vi "E727_StageNavigatorModule.vi"(0 "Up Z x4":bool, 1 "Up Z x2":bool, 2 "Up Z":bool, 3 "StageChannels":string[](array[string]), 4 "Up x4":bool, 5 "Up x2":bool, 6 "Up":bool, 7 "Up x0.5":bool, 8 "Right x0.5":bool, 9 "Left x0.5":bool, 10 "Right":bool, 11 "Left":bool, 12 "Right x2":bool, 13 "Left x2":bool, 14 "Right x4":bool, 15 "Left x4":bool, 17 "X / Y Resolution (um)":dbl=10.0 min=1.0, 19 "Z Resolution (um)":dbl=30.0 min=1.0, 20 "Down Z x4":bool, 21 "Down Z x2":bool, 22 "Down Z":bool, 23 "stop":bool, 24 "Down x4":bool, 25 "Down x2":bool, 26 "Down":bool, 27 "Down x0.5":bool) -> (16 "Position":dbl[](array[numeric]) format="%.6f")   [LabVIEW 2022 SP3]
panel:
  in  "Repeats":dbl=1.0 min=1.0
  # "STAGE"
  # "Z Focus"
  # "X / Y Navigation"
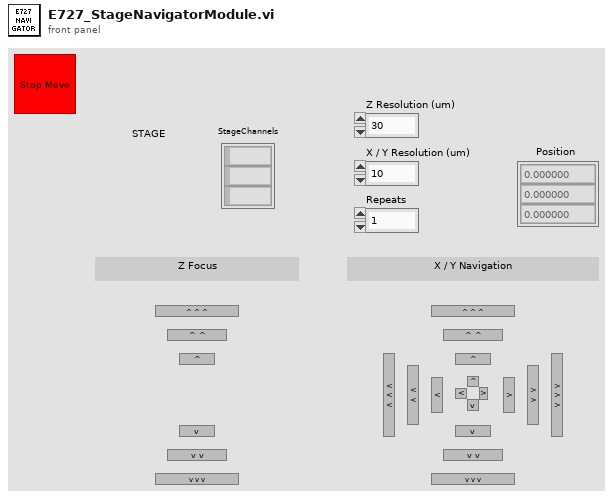
[diagram p1: front panel]
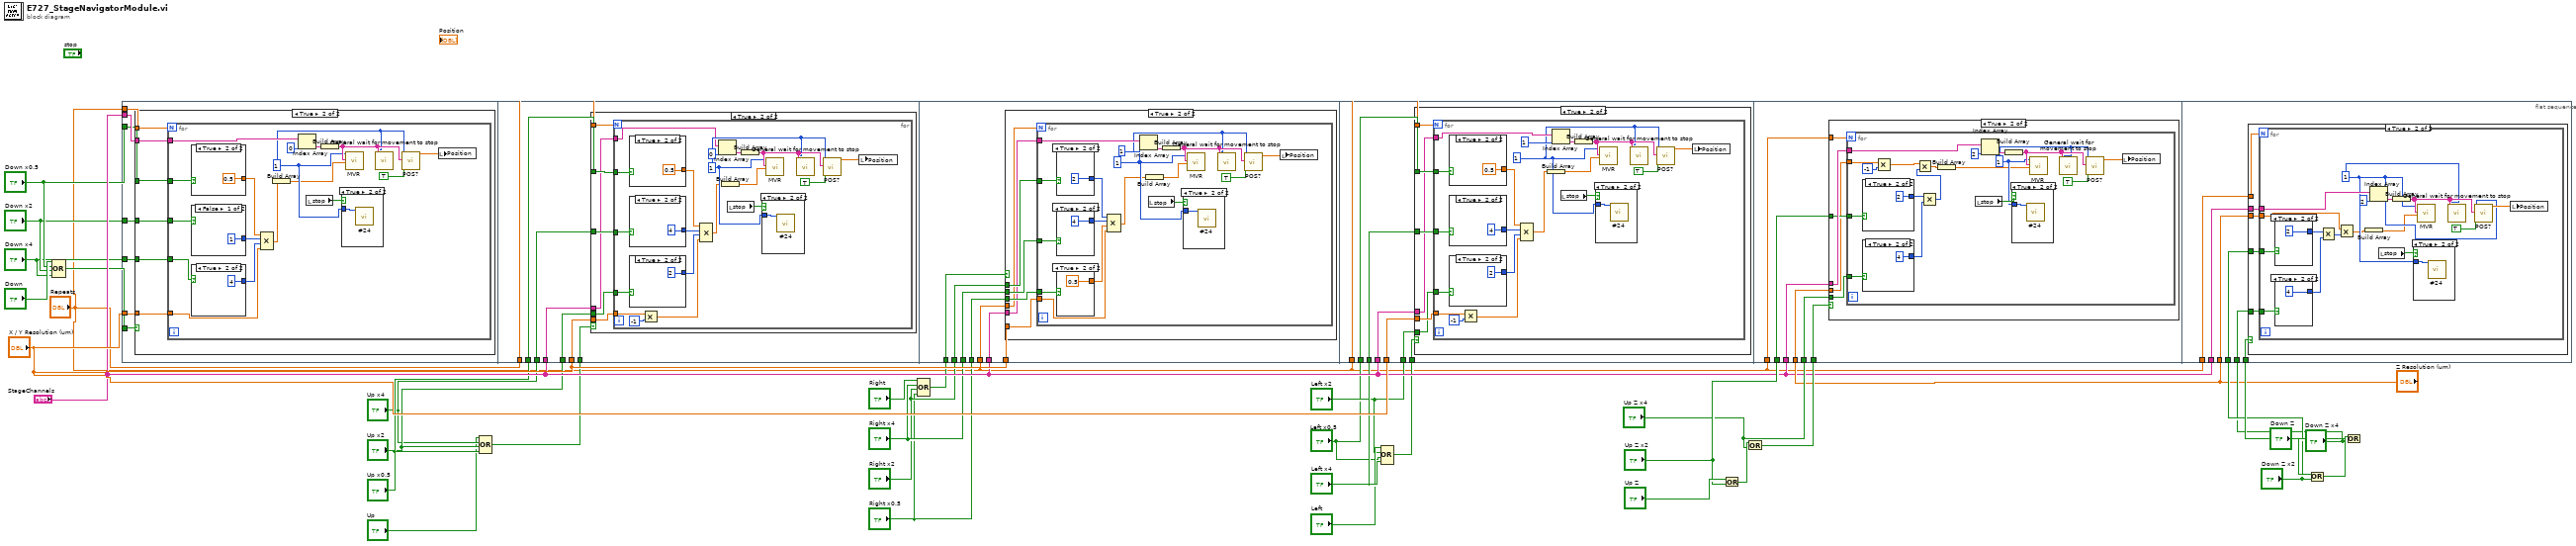
[diagram p0: block diagram]
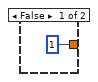
[diagram p4: hidden frame]
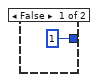
[diagram p5: hidden frame]
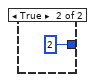
[diagram p6: hidden frame]
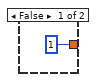
[diagram p9: hidden frame]
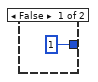
[diagram p10: hidden frame]
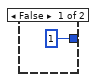
[diagram p11: hidden frame]
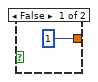
[diagram p14: hidden frame]
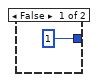
[diagram p15: hidden frame]
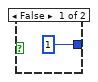
[diagram p16: hidden frame]
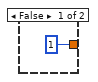
[diagram p19: hidden frame]
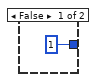
[diagram p20: hidden frame]
diagram:
  n1 = Compound Arithmetic op=OR("Down", "Down x0.5", "Down x2", "Down x4") -> (w6:bool)
  n2 = flat-sequence {
    tunnel: "X / Y Resolution (um)" -> [w40]
    tunnel: "StageChannels" -> [w41]
    tunnel: w6 -> [w39]
    tunnel: "Down x2" -> [w38]
    tunnel: "Down x4" -> [w37]
    tunnel: "Down x0.5" -> [w36]
    tunnel: "Repeats" -> [w35]
    tunnel: "X / Y Resolution (um)" -> [w78]
    tunnel: "StageChannels" -> [w77]
    tunnel: "Up x2" -> [w76]
    tunnel: w11 -> [w75]
    tunnel: "Up x4" -> [w74]
    tunnel: "Up x0.5" -> [w73]
    tunnel: "Repeats" -> [w72]
    tunnel: "StageChannels" -> [w117]
    tunnel: "Right x2" -> [w116]
    tunnel: "Right x4" -> [w115]
    tunnel: "X / Y Resolution (um)" -> [w114]
    tunnel: w21 -> [w113]
    tunnel: "Right x0.5" -> [w112]
    tunnel: "Repeats" -> [w111]
    tunnel: "StageChannels" -> [w154]
    tunnel: "X / Y Resolution (um)" -> [w153]
    tunnel: w16 -> [w152]
    tunnel: "Left x4" -> [w151]
    tunnel: "Left x2" -> [w150]
    tunnel: "Left x0.5" -> [w149]
    tunnel: "Repeats" -> [w148]
    tunnel: "StageChannels" -> [w192]
    tunnel: "Z Resolution (um)" -> [w191]
    tunnel: w32 -> [w190]
    tunnel: "Up Z x2" -> [w189]
    tunnel: "Up Z x4" -> [w188]
    tunnel: "Repeats" -> [w187]
    tunnel: "StageChannels" -> [w226]
    tunnel: "Z Resolution (um)" -> [w225]
    tunnel: w26 -> [w224]
    tunnel: "Down Z x2" -> [w223]
    tunnel: "Down Z x4" -> [w222]
    tunnel: "Repeats" -> [w221]
    frame #0 {
      n3 = case shown="True" w39 {
        tunnel: w40 -> [_ w44]
        tunnel: w41 -> [_ w47]
        tunnel: w38 -> [_ w46]
        tunnel: w37 -> [_ w45]
        tunnel: w36 -> [_ w43]
        tunnel: w35 -> [_ w42]
        frame False {
        }
        frame True {
          n4 = for {
            N: w42 -> [_]
            tunnel: w47 -> [w51]
            tunnel: w46 -> [w64]
            tunnel: w45 -> [w63]
            tunnel: w44 -> [w62]
            tunnel: w43 -> [w58]
            w50 = 1 ("System no.")
            n5 = case shown="True" w58 {
              tunnel: [1 0.5] -> w61
              frame False {
              }
              frame True {
              }
            }
            n6 = case shown="False" w64 {
              tunnel: [1 2] -> w59
              frame False {
              }
              frame True {
              }
            }
            n7 = case shown="True" w63 {
              tunnel: [1 4] -> w60
              frame False {
              }
              frame True {
              }
            }
            n8 = Compound Arithmetic op=MULTIPLY(w61, w59, w60, w62) -> (w49:dbl)
            n9 = Build Array(w49) -> (w48:dbl[])
            n10 = Index Array(array=w51, index=0) -> (element=w54:string)
            n11 = local read "stop"() -> (w55:bool)
            n12 = Build Array(w54) -> (w56:string[])
            n13 = case shown="True" w55 {
              tunnel: w50 -> [_ w65]
              frame False {
              }
              frame True {
                n14 = call "#24.vi"("System no."=w65) -> ()  [unwired: 1 in, 18 out]
              }
            }
            n15 = call "MVR.vi"("System no."=w50, "Axes to move"=w56, "Position values"=w48) -> ()  [unwired: 2 in, 15 out]
            n16 = call "General wait for movement to stop.vi"("System no."=w50, "Axes to wait for"=w56) -> ()  [unwired: 6 in, 12 out]
            n17 = call "POS?.vi"("System no."=w50, "Axes to query"=w56, "All axes?"=TRUE) -> ("Position"=w57:dbl[])  [unwired: 2 in, 14 out]
            n18 = local write "Position"(w57) -> ()
          }
        }
      }
    }
    frame #1 {
      n19 = case shown="True" w75 {
        tunnel: w78 -> [_ w84]
        tunnel: w77 -> [_ w80]
        tunnel: w76 -> [_ w83]
        tunnel: w74 -> [_ w82]
        tunnel: w73 -> [_ w81]
        tunnel: w72 -> [_ w79]
        frame False {
        }
        frame True {
          n20 = for {
            N: w79 -> [_]
            tunnel: w84 -> [w95]
            tunnel: w83 -> [w102]
            tunnel: w82 -> [w101]
            tunnel: w81 -> [w96]
            tunnel: w80 -> [w87]
            w88 = 1 ("System no.")
            n21 = case shown="True" w96 {
              tunnel: [1 0.5] -> w99
              frame False {
              }
              frame True {
              }
            }
            n22 = case shown="True" w101 {
              tunnel: [1 4] -> w98
              frame False {
              }
              frame True {
              }
            }
            n23 = case shown="True" w102 {
              tunnel: [1 2] -> w97
              frame False {
              }
              frame True {
              }
            }
            n24 = Multiply(x=w95, y=-1) -> (x*y=w100:dbl)
            n25 = Compound Arithmetic op=MULTIPLY(w99, w98, w97, w100) -> (w85:dbl)
            n26 = Index Array(array=w87, index=0) -> (element=w91:string)
            n27 = Build Array(w85) -> (w86:dbl[])
            n28 = local read "stop"() -> (w92:bool)
            n29 = Build Array(w91) -> (w93:string[])
            n30 = case shown="True" w92 {
              tunnel: w88 -> [_ w104]
              frame False {
              }
              frame True {
                n31 = call "#24.vi"("System no."=w104) -> ()  [unwired: 1 in, 18 out]
              }
            }
            n32 = call "MVR.vi"("System no."=w88, "Axes to move"=w93, "Position values"=w86) -> ()  [unwired: 2 in, 15 out]
            n33 = call "General wait for movement to stop.vi"("System no."=w88, "Axes to wait for"=w93) -> ()  [unwired: 6 in, 12 out]
            n34 = call "POS?.vi"("System no."=w88, "Axes to query"=w93, "All axes?"=TRUE) -> ("Position"=w94:dbl[])  [unwired: 2 in, 14 out]
            n35 = local write "Position"(w94) -> ()
          }
        }
      }
    }
    frame #2 {
      n36 = case shown="True" w113 {
        tunnel: w114 -> [_ w120]
        tunnel: w117 -> [_ w119]
        tunnel: w116 -> [_ w123]
        tunnel: w115 -> [_ w122]
        tunnel: w112 -> [_ w121]
        tunnel: w111 -> [_ w118]
        frame False {
        }
        frame True {
          n37 = for {
            N: w118 -> [_]
            tunnel: w123 -> [w140]
            tunnel: w122 -> [w139]
            tunnel: w121 -> [w137]
            tunnel: w120 -> [w134]
            tunnel: w119 -> [w128]
            w126 = 1 ("System no.")
            n38 = case shown="True" w140 {
              tunnel: [1 2] -> w136
              frame False {
              }
              frame True {
              }
            }
            n39 = case shown="True" w139 {
              tunnel: [1 4] -> w135
              frame False {
              }
              frame True {
              }
            }
            n40 = case shown="True" w137 {
              tunnel: [1 0.5] -> w138
              frame False {
              }
              frame True {
              }
            }
            n41 = Compound Arithmetic op=MULTIPLY(w136, w135, w138, w134) -> (w124:dbl)
            n42 = Index Array(array=w128, index=1) -> (element=w130:string)
            n43 = Build Array(w124) -> (w125:dbl[])
            n44 = local read "stop"() -> (w131:bool)
            n45 = Build Array(w130) -> (w132:string[])
            n46 = case shown="True" w131 {
              tunnel: w126 -> [_ w141]
              frame False {
              }
              frame True {
                n47 = call "#24.vi"("System no."=w141) -> ()  [unwired: 1 in, 18 out]
              }
            }
            n48 = call "MVR.vi"("System no."=w126, "Axes to move"=w132, "Position values"=w125) -> ()  [unwired: 2 in, 15 out]
            n49 = call "General wait for movement to stop.vi"("System no."=w126, "Axes to wait for"=w132) -> ()  [unwired: 6 in, 12 out]
            n50 = call "POS?.vi"("System no."=w126, "Axes to query"=w132, "All axes?"=TRUE) -> ("Position"=w133:dbl[])  [unwired: 2 in, 14 out]
            n51 = local write "Position"(w133) -> ()
          }
        }
      }
    }
    frame #3 {
      n52 = case shown="True" w152 {
        tunnel: w153 -> [_ w160]
        tunnel: w154 -> [_ w156]
        tunnel: w150 -> [_ w159]
        tunnel: w151 -> [_ w158]
        tunnel: w149 -> [_ w157]
        tunnel: w148 -> [_ w155]
        frame False {
        }
        frame True {
          n53 = for {
            N: w155 -> [_]
            tunnel: w160 -> [w179]
            tunnel: w159 -> [w177]
            tunnel: w158 -> [w176]
            tunnel: w157 -> [w171]
            tunnel: w156 -> [w164]
            w163 = 1 ("System no.")
            n54 = case shown="True" w171 {
              tunnel: [1 0.5] -> w175
              frame False {
              }
              frame True {
              }
            }
            n55 = case shown="True" w176 {
              tunnel: [1 4] -> w173
              frame False {
              }
              frame True {
              }
            }
            n56 = case shown="True" w177 {
              tunnel: [1 2] -> w172
              frame False {
              }
              frame True {
              }
            }
            n57 = Multiply(x=w179, y=-1) -> (x*y=w174:dbl)
            n58 = Compound Arithmetic op=MULTIPLY(w175, w173, w172, w174) -> (w161:dbl)
            n59 = Build Array(w161) -> (w162:dbl[])
            n60 = Index Array(array=w164, index=1) -> (element=w167:string)
            n61 = local read "stop"() -> (w168:bool)
            n62 = Build Array(w167) -> (w169:string[])
            n63 = case shown="True" w168 {
              tunnel: w163 -> [_ w180]
              frame False {
              }
              frame True {
                n64 = call "#24.vi"("System no."=w180) -> ()  [unwired: 1 in, 18 out]
              }
            }
            n65 = call "MVR.vi"("System no."=w163, "Axes to move"=w169, "Position values"=w162) -> ()  [unwired: 2 in, 15 out]
            n66 = call "General wait for movement to stop.vi"("System no."=w163, "Axes to wait for"=w169) -> ()  [unwired: 6 in, 12 out]
            n67 = call "POS?.vi"("System no."=w163, "Axes to query"=w169, "All axes?"=TRUE) -> ("Position"=w170:dbl[])  [unwired: 2 in, 14 out]
            n68 = local write "Position"(w170) -> ()
          }
        }
      }
    }
    frame #4 {
      n69 = case shown="True" w190 {
        tunnel: w191 -> [_ w194]
        tunnel: w192 -> [_ w197]
        tunnel: w189 -> [_ w196]
        tunnel: w188 -> [_ w195]
        tunnel: w187 -> [_ w193]
        frame False {
        }
        frame True {
          n70 = for {
            N: w193 -> [_]
            tunnel: w197 -> [w201]
            tunnel: w196 -> [w212]
            tunnel: w195 -> [w211]
            tunnel: w194 -> [w208]
            w200 = 1 ("System no.")
            n71 = case shown="True" w212 {
              tunnel: [1 2] -> w214
              frame False {
              }
              frame True {
              }
            }
            n72 = case shown="True" w211 {
              tunnel: [1 4] -> w215
              frame False {
              }
              frame True {
              }
            }
            n73 = Multiply(x=w208, y=-1) -> (x*y=w209:dbl)
            n74 = Multiply(x=w214, y=w215) -> (x*y=w213:i32)
            n75 = Multiply(x=w209, y=w213) -> (x*y=w199:dbl)
            n76 = Build Array(w199) -> (w198:dbl[])
            n77 = local read "stop"() -> (w205:bool)
            n78 = Index Array(array=w201, index=2) -> (element=w204:string)
            n79 = Build Array(w204) -> (w206:string[])
            n80 = case shown="True" w205 {
              tunnel: w200 -> [_ w216]
              frame False {
              }
              frame True {
                n81 = call "#24.vi"("System no."=w216) -> ()  [unwired: 1 in, 18 out]
              }
            }
            n82 = call "MVR.vi"("System no."=w200, "Axes to move"=w206, "Position values"=w198) -> ()  [unwired: 2 in, 15 out]
            n83 = call "General wait for movement to stop.vi"("System no."=w200, "Axes to wait for"=w206) -> ()  [unwired: 6 in, 12 out]
            n84 = call "POS?.vi"("System no."=w200, "Axes to query"=w206, "All axes?"=TRUE) -> ("Position"=w207:dbl[])  [unwired: 2 in, 14 out]
            n85 = local write "Position"(w207) -> ()
          }
        }
      }
    }
    frame #5 {
      n86 = case shown="True" w224 {
        tunnel: w225 -> [_ w230]
        tunnel: w226 -> [_ w231]
        tunnel: w223 -> [_ w229]
        tunnel: w222 -> [_ w228]
        tunnel: w221 -> [_ w227]
        frame False {
        }
        frame True {
          n87 = for {
            N: w227 -> [_]
            tunnel: w231 -> [w235]
            tunnel: w230 -> [w244]
            tunnel: w229 -> [w243]
            tunnel: w228 -> [w242]
            w234 = 1 ("System no.")
            n88 = case shown="True" w243 {
              tunnel: [1 2] -> w246
              frame False {
              }
              frame True {
              }
            }
            n89 = case shown="True" w242 {
              tunnel: [1 4] -> w247
              frame False {
              }
              frame True {
              }
            }
            n90 = Multiply(x=w246, y=w247) -> (x*y=w245:i32)
            n91 = Multiply(x=w244, y=w245) -> (x*y=w233:dbl)
            n92 = Build Array(w233) -> (w232:dbl[])
            n93 = Index Array(array=w235, index=2) -> (element=w238:string)
            n94 = local read "stop"() -> (w239:bool)
            n95 = Build Array(w238) -> (w240:string[])
            n96 = case shown="True" w239 {
              tunnel: w234 -> [_ w248]
              frame False {
              }
              frame True {
                n97 = call "#24.vi"("System no."=w248) -> ()  [unwired: 1 in, 18 out]
              }
            }
            n98 = call "MVR.vi"("System no."=w234, "Axes to move"=w240, "Position values"=w232) -> ()  [unwired: 2 in, 15 out]
            n99 = call "General wait for movement to stop.vi"("System no."=w234, "Axes to wait for"=w240) -> ()  [unwired: 6 in, 12 out]
            n100 = call "POS?.vi"("System no."=w234, "Axes to query"=w240, "All axes?"=TRUE) -> ("Position"=w241:dbl[])  [unwired: 2 in, 14 out]
            n101 = local write "Position"(w241) -> ()
          }
        }
      }
    }
  }
  n102 = Compound Arithmetic op=OR("Up", "Up x4", "Up x2", "Up x0.5") -> (w11:bool)
  n103 = Compound Arithmetic op=OR("Right", "Right x4", "Right x2", "Right x0.5") -> (w21:bool)
  n104 = Compound Arithmetic op=OR("Left", "Left x2", "Left x0.5", "Left x4") -> (w16:bool)
  n105 = Or(x="Up Z", y="Up Z x2") -> (x .or. y?=w34:bool)
  n106 = Or(x=w34, y="Up Z x4") -> (x .or. y?=w32:bool)
  n107 = Or(x="Down Z", y="Down Z x2") -> (x .or. y?=w28:bool)
  n108 = Or(x=w28, y="Down Z x4") -> (x .or. y?=w26:bool)
